vi "testTrigMatrix.vi"() -> ()   [LabVIEW 2017]
uses:
  <instrlib>/niDMM/nidmm.llb/niDMM Powerline Frequency.ctl
  <instrlib>/niDMM/nidmm.llb/niDMM Resolution in Digits.ctl
  <instrlib>/niDMM/nidmm.llb/niDMM Function.ctl
  <instrlib>/niDMM/nidmm.llb/niDMM Auto Zero.ctl
  <instrlib>/niDMM/nidmm.llb/niDMM ADC Calibration.ctl
  <instrlib>/niDMM/nidmm.llb/niDMM Configure Measurement Absolute.vi
panel:
  out "Measurement":dbl format="%.5f"
  out "Route Specification":string
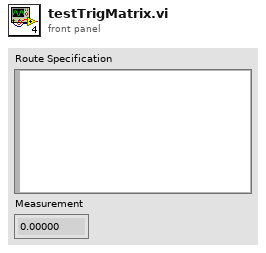
[diagram p1: front panel]
types:
  T1 = typedef "niDMM ADC Calibration.ctl" = i32
  T2 = typedef "niDMM Auto Zero.ctl" = i32
  T3 = typedef "niDMM Function.ctl" = enum16{"DC Volts", "AC Volts", "DC Current", "AC Current", "2-wire Resistance", "4-wire Resistance", "Diode", "Frequency", "Period", "AC Volts DC Coupled", "Capacitance", "Inductance", "Temperature"}
  T4 = typedef "niDMM Resolution in Digits.ctl" = dbl
  T5 = typedef "niDMM Powerline Frequency.ctl" = enum16{"60 Hz", "50 Hz"}
  T6 = typedef "niSE SessionRefnum.ctl" = refnum<k1>
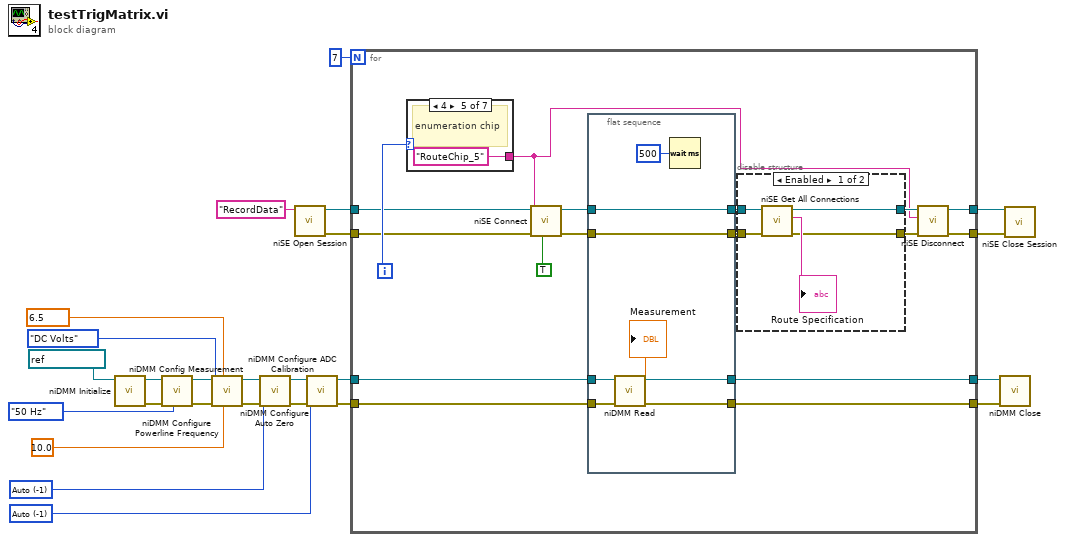
[diagram p0: block diagram]
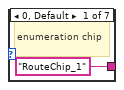
[diagram p2: hidden frame]
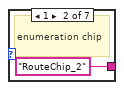
[diagram p3: hidden frame]
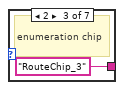
[diagram p4: hidden frame]
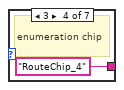
[diagram p5: hidden frame]
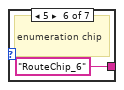
[diagram p6: hidden frame]
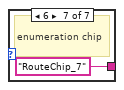
[diagram p7: hidden frame]
diagram:
  w8 = T1 -1 items=["Auto"=-1, "Off"=0, "On"=1] ("ADC Calibration")
  w11 = T2 -1 items=["Auto"=-1, "Off"=0, "On"=1, "Once"=2] ("Auto Zero")
  w15 = T4 6.5 items=["3 1/2"=3.5, "4 1/2"=4.5, "5 1/2"=5.5, "6 1/2"=6.5, "7 1/2"=7.5] ("Resolution in Digits")
  n1 = call <instrlib>:"niDMM Initialize.vi"("Instrument Descriptor"=refnum<k15> "PXI1Slot2") -> ("error out"=w20:errorcluster, "instrument handle out"=w19:refnum<k15>)  [unwired: 9 in]
  n2 = call <instrlib>:"niDMM Configure Powerline Frequency.vi"("Powerline Frequency"=niDMM_Powerline_Frequency."50 Hz", "error in (no error)"=w20, "instrument handle"=w19) -> ("error out"=w16:errorcluster, "instrument handle out"=w17:refnum<k15>)  [unwired: 7 in]
  n3 = call-poly <instrlib>:"niDMM Config Measurement.vi"("Range"=10.0, "Resolution"=w15, "error in (no error)"=w16, "Function"=niDMM_Function."DC Volts", "instrument handle"=w17) -> ("error out"=w13:errorcluster, "instrument handle out"=w12:refnum<k15>)  [unwired: 5 in]
  n4 = call <instrlib>:"niDMM Configure Auto Zero.vi"("error in (no error)"=w13, "Auto Zero"=w11, "instrument handle"=w12) -> ("error out"=w10:errorcluster, "instrument handle out"=w9:refnum<k15>)  [unwired: 7 in]
  n5 = call <vilib>:"niSE Open Session.vi"("Virtual Device Name (SwitchConfiguration1)"="RecordData") -> ("error out"=w23:errorcluster, "NISE Session (out)"=w22:T6)  [unwired: 5 in]
  n6 = call <instrlib>:"niDMM Configure ADC Calibration.vi"("error in (no error)"=w10, "ADC Calibration"=w8, "instrument handle"=w9) -> ("error out"=w7:errorcluster, "instrument handle out"=w6:refnum<k15>)  [unwired: 7 in]
  n7 = for {
    N: 7 -> [_]
    tunnel: w23 -> [w40]
    tunnel: w22 -> [w39]
    tunnel: w7 -> [w34]
    tunnel: w6 -> [w33]
    tunnel: [w32] -> w5
    tunnel: [w31] -> w4
    tunnel: [w27] -> w3
    tunnel: [w28] -> w2
    i -> [w41]
    n8 = case shown="4" w41 {
      tunnel: ["RouteChip_1" ("Connection Specification (\"\")") "RouteChip_2" ("Connection Specification (\"\")") "RouteChip_3" ("Connection Specification (\"\")") "RouteChip_4" ("Connection Specification (\"\")") "RouteChip_5" ("Connection Specification (\"\")") "RouteChip_6" ("Connection Specification (\"\")") "RouteChip_7" ("Connection Specification (\"\")")] -> w26
      frame 0, Default {
        # "enumeration chip"
      }
      frame 1 {
        # "enumeration chip"
      }
      frame 2 {
        # "enumeration chip"
      }
      frame 3 {
        # "enumeration chip"
      }
      frame 4 {
        # "enumeration chip"
      }
      frame 5 {
        # "enumeration chip"
      }
      frame 6 {
        # "enumeration chip"
      }
    }
    n9 = call <vilib>:"niSE Connect.vi"("Wait For Debounce (T)"=TRUE, "error in (no error)"=w40, "Connection Specification (\"\")"=w26, "NISE Session (in)"=w39) -> ("error out"=w35:errorcluster, "NISE Session (out)"=w37:T6)  [unwired: 6 in]
    n10 = flat-sequence {
      tunnel: [w50] -> w38
      tunnel: w37 -> [w50]
      tunnel: [w49] -> w36
      tunnel: w35 -> [w49]
      tunnel: w34 -> [w48]
      tunnel: w33 -> [w47]
      tunnel: [w46] -> w32
      tunnel: [w45] -> w31
      frame #0 {
        n11 = call <instrlib>:"niDMM Read.vi"("error in (no error)"=w48, "instrument handle"=w47) -> ("error out"=w45:errorcluster, "Measurement"=→"Measurement":dbl, "instrument handle out"=w46:refnum<k15>)  [unwired: 7 in]
        n12 = Wait (ms)(milliseconds to wait=u32 500) -> ()  [unwired: 1 out]
      }
    }
    n13 = disable-structure shown="Enabled" {
      disable-tunnel: w36 -> [w62 w63]
      disable-tunnel: w38 -> [w61 w64]
      disable-tunnel: [w59 w63] -> w30
      disable-tunnel: [w58 w64] -> w29
      frame Enabled {
        n14 = call <vilib>:"niSE Get All Connections.vi"("error in (no error)"=w62, "NISE Session (in)"=w61) -> ("error out"=w59:errorcluster, "Route Specification"=→"Route Specification":string, "NISE Session (out)"=w58:T6)  [unwired: 3 in]
      }
      frame Disabled {
      }
    }
    n15 = call <vilib>:"niSE Disconnect.vi"("error in (no error)"=w30, "Disconnection Specification (\"\")"=w26, "NISE Session (in)"=w29) -> ("error out"=w27:errorcluster, "NISE Session (out)"=w28:T6)  [unwired: 3 in]
  }
  n16 = call <instrlib>:"niDMM Close.vi"("error in (no error)"=w4, "instrument handle"=w5) -> ()  [unwired: 9 in, 1 out]
  n17 = call <vilib>:"niSE Close Session.vi"("error in (no error)"=w3, "NISE Session (in)"=w2) -> ()  [unwired: 5 in, 1 out]
